vi "Transportation Problem using Linear Programming.vi"(9 "Transport Costs":dbl[][](array[numeric]), 10 "Traders":cluster{"name":string, "produced units":dbl}[](array[cluster]), 11 "Producers":cluster{"name":string, "produced units":dbl}[](array[cluster])) -> (0 "error":i32, 2 "minimal cost":dbl, 3 "Solution":dbl[][](array[numeric]))   [LabVIEW 2023]
doc: "Prepare the data in the Transportation Problem format to solve using the Linear Programming matrices (C,M,B)."
uses:
  <vilib>/gmath/NI_Gmath.lvlib
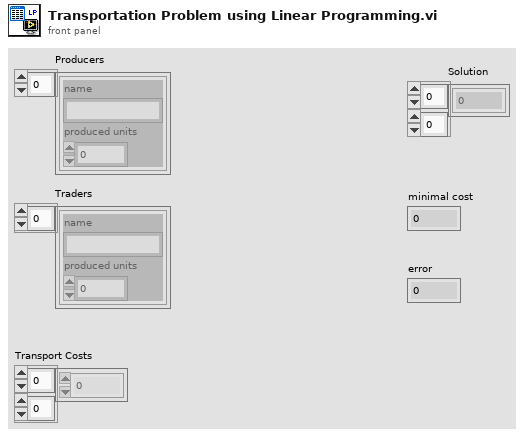
[diagram p1: front panel]
types:
  T1 = typedef "NI_Matrix.lvlib/RealMatrix.ctl" = dbl[][]
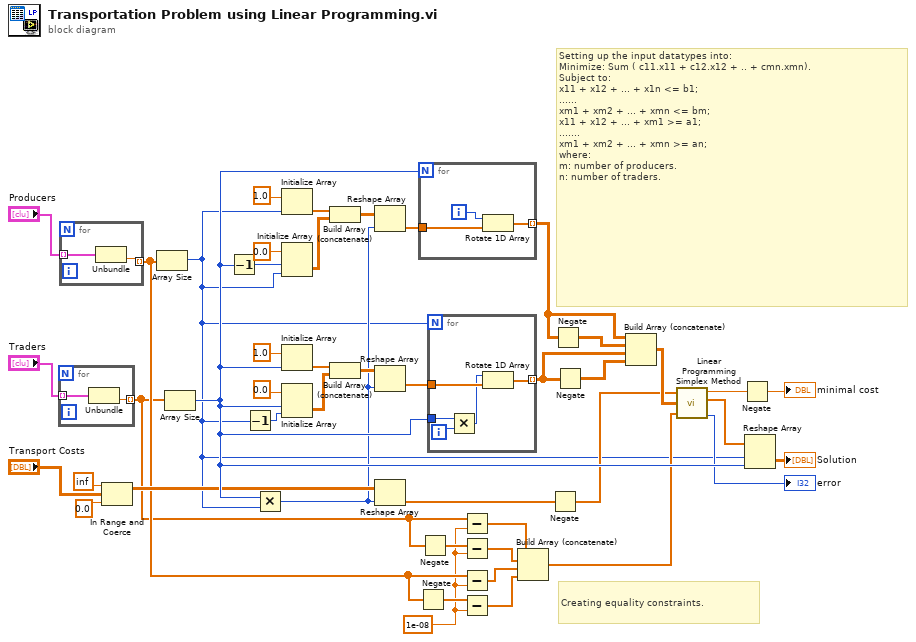
[diagram p0: block diagram]
diagram:
  w1 = 1e-08
  # "Setting up the input datatypes into:\nMinimize: Sum ( c11.x11 + c12.x12 + .. + cmn.xmn).\nSubject to:\nx11 + x12 + ... + x1n <= b1;\n......\nxm1 + xm2 + ... + xmn <= bm;\nx11 + x12 + ... + xm1 >= a1;\n.......\nxm1 + xm2 + ... + xmn >= an;\nwhere:\nm: number of producers.\nn: number of traders."
  # "Creating equality constraints."
  n1 = for {
    tunnel: "Traders" -> [w47] mode=indexing
    tunnel: [w46] -> w10 mode=indexing
    n2 = Unbundle(w47) -> ("produced units"=w46:dbl)  [unwired: 1 out]
  }
  n3 = for {
    tunnel: "Producers" -> [w49] mode=indexing
    tunnel: [w48] -> w11 mode=indexing
    n4 = Unbundle(w49) -> ("produced units"=w48:dbl)  [unwired: 1 out]
  }
  n5 = In Range and Coerce(upper limit=inf, x="Transport Costs", lower limit=0.0) -> (coerced(x)=w13:dbl[][])  [unwired: 1 out]
  n6 = Array Size(array=w11) -> (size(s)=w3:i32)
  n7 = Array Size(array=w10) -> (size(s)=w44:i32)
  n8 = Decrement(x=w44) -> (x-1=w32:i32)
  n9 = Decrement(x=w3) -> (x-1=w25:i32)
  n10 = Multiply(x=w44, y=w3) -> (x*y=w5:i32)
  n11 = Initialize Array(1.0, w3) -> (w37:dbl[])
  n12 = Initialize Array(0.0, w32, w3) -> (w31:dbl[][])
  n13 = Initialize Array(1.0, w44) -> (w26:dbl[])
  n14 = Initialize Array(0.0, w44, w25) -> (w27:dbl[][])
  n15 = Build Array (concatenate)(w37, w31) -> (w12:T1)
  n16 = Build Array (concatenate)(w26, w27) -> (w28:T1)
  n17 = Reshape Array(w12, w5) -> (w30:dbl[])
  n18 = Reshape Array(w28, w5) -> (w29:dbl[])
  n19 = Reshape Array(w13, w5) -> (w39:dbl[])
  n20 = Negate(x=w11) -> (-x=w17:dbl[])
  n21 = for {
    N: w44 -> [_]
    tunnel: w30 -> [w52]
    tunnel: [w51] -> w33 mode=indexing
    i -> [w50]
    n22 = Rotate 1D Array(1:w52, 2:w50) -> (0:w51:dbl[])
  }
  n23 = Negate(x=w10) -> (-x=w20:dbl[])
  n24 = for {
    N: w3 -> [_]
    tunnel: w29 -> [w57]
    tunnel: w44 -> [w56]
    tunnel: [w55] -> w35 mode=indexing
    i -> [w54]
    n25 = Multiply(x=w56, y=w54) -> (x*y=w53:i32)
    n26 = Rotate 1D Array(1:w57, 2:w53) -> (0:w55:dbl[])
  }
  n27 = Subtract(x=w10, y=w1) -> (x-y=w19:dbl[])
  n28 = Subtract(x=w20, y=w1) -> (x-y=w18:dbl[])
  n29 = Subtract(x=w11, y=w1) -> (x-y=w16:dbl[])
  n30 = Subtract(x=w17, y=w1) -> (x-y=w15:dbl[])
  n31 = Build Array (concatenate)(w19, w18, w16, w15) -> (w38:dbl[])
  n32 = Negate(x=w39) -> (-x=w40:dbl[])
  n33 = Negate(x=w33) -> (-x=w34:dbl[][])
  n34 = Negate(x=w35) -> (-x=w36:dbl[][])
  n35 = Build Array (concatenate)(w33, w34, w35, w36) -> (w42:dbl[][])
  n36 = call <vilib>:"Linear Programming Simplex Method.vi"("C"=w40, "M"=w42, "B"=w38) -> ("maximum"=w41:dbl, "X"=w43:dbl[], "error"=→"error":i32)  [unwired: 1 out]
  n37 = Negate(x=w41) -> (-x=→"minimal cost":dbl)
  n38 = Reshape Array(w43, w3, w44) -> (→"Solution":dbl[][])
